vi "test reset.vi"   [LabVIEW 2018]
uses:
  <vilib>/rvi/interface/nirviReadWriteControl/nirviReadWriteControl.xnode
  <vilib>/rvi/interface/Simulation/niFpgaSimulationCallBeginRW.vi
  <vilib>/rvi/errors/niLvFpgaAdjustHostInterfaceError.vi
  <vilib>/rvi/interface/nirviOpenFPGA/nirviOpenFPGA.xnode
  NiFpgaLv.dll
  <vilib>/Utility/error.llb/Error Cluster From Error Code.vi
  FPGA Bitfiles/Dentalrobot_FPGATarget_1DIOBoardTestFPG_3A5PBD8+om0.lvbitx
  FPGA/FPGA_Dental robot.vi
  <vilib>/FPGAPlugInAG/myRIO-1900/niLvFpga_Open_myRIO-1900.vi
  <vilib>/rvi/interface/common/dynamic/niFpgaDynamicAddResources.vi
  <vilib>/platform/TimedLoop/XDataNode/XDataNode.xnode
  <vilib>/Platform/TimedLoop/XDataNode/nitl_modes.ctl
  <vilib>/Platform/TimedLoop/XDataNode/XDNodeRunTimeDep.lvlib
  <vilib>/Platform/TimedLoop/XDataNode/wakeup.ctl
  <vilib>/Platform/TimedLoop/XDataNode/timing_clust.ctl
panel:
  # "Servor"
  # "Stepper"
types:
  T1 = typedef "XDNodeRunTimeDep.lvlib/timing_clust.ctl" = cluster{"Expected End [f-1]":u64, "Actual End [f-1]":u64, "Finished Late? [f-1]":bool, "Expected End [i-1]":u64, "Actual End [i-1]":u64, "Finished Late? [i-1]":bool, "Expected Start [i]":u64, "Actual Start [i]":u64, "Expected Start [f]":u64, "Actual Start [f]":u64, "Source Name":string, "Structure Name":string, "Period":i64, "Deadline":i64, "Offset":i64, "Start":i64, "Priority":i32, "Timeout":i32, "Mode":T2, "Wakeup Reason":T3, "Error":errorcluster, "Source Type":string, "Secondary Source Type":string, "Global End Time":u64, "Global Start Time":u64, "Frame Duration":u64, "Iteration Duration":u64, "Assigned CPU":i32, "I/O Scan Engine Mode":u32}
  T2 = typedef "XDNodeRunTimeDep.lvlib/nitl_modes.ctl" = enum32{"No Change", "Process missed periods, maintain original phase", "Discard missed periods, maintain original phase", "Process missed periods, ignore original phase", "Discard missed periods, ignore original phase"}
  T3 = typedef "XDNodeRunTimeDep.lvlib/wakeup.ctl" = enum32{"Normal", "Aborted", "Asynchronous wakeup", "Timing source error", "Timed loop error", "Timeout"}
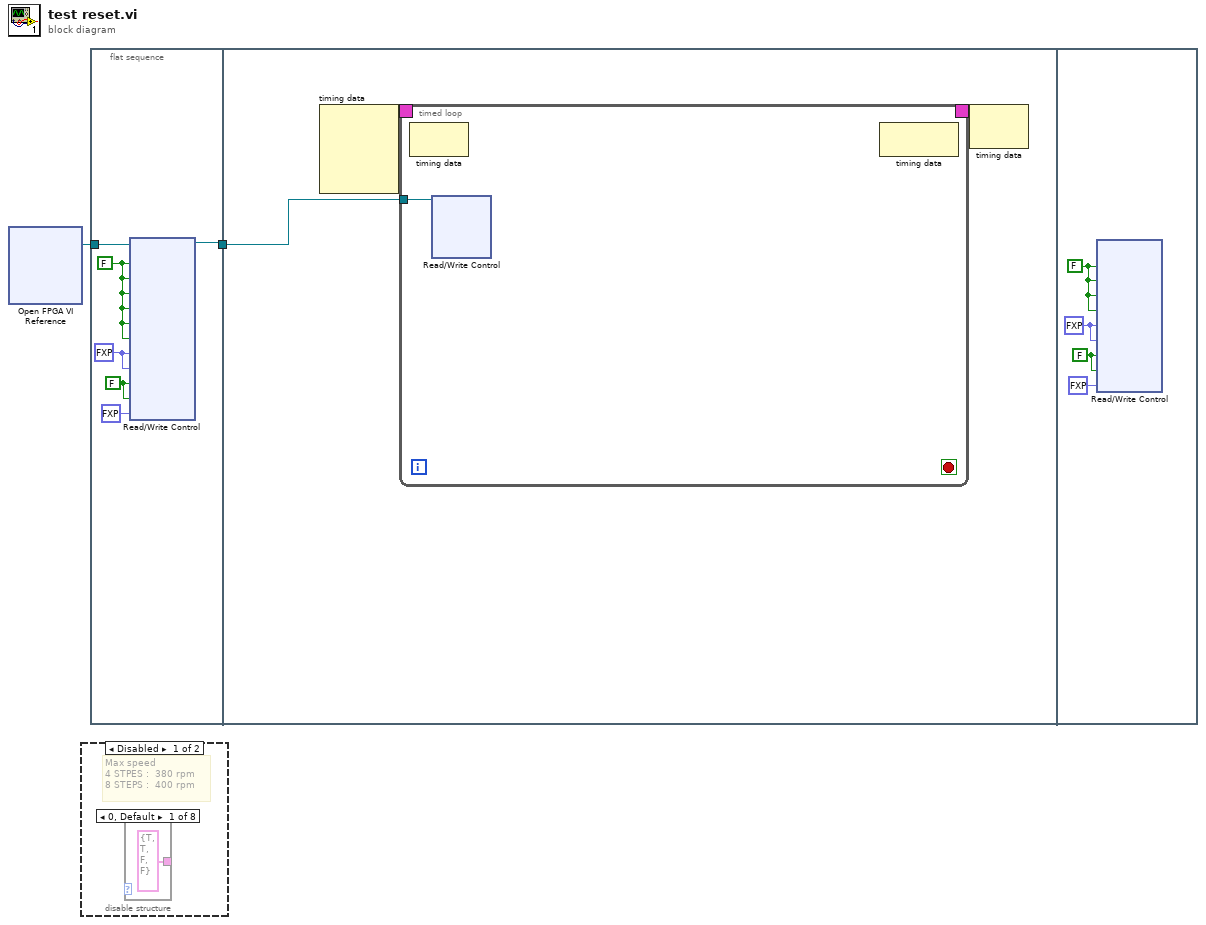
[diagram p0: block diagram]
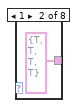
[diagram p2: hidden frame]
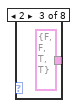
[diagram p3: hidden frame]
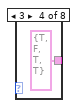
[diagram p4: hidden frame]
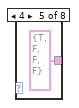
[diagram p5: hidden frame]
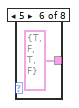
[diagram p6: hidden frame]
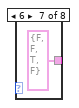
[diagram p7: hidden frame]
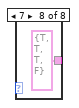
[diagram p8: hidden frame]
diagram:
  n1 = xnode "Open FPGA VI Reference"() -> ("FPGA VI Reference Out"=w1:refnum<k20>)  [unwired: 2 in, 1 out]
  n2 = disable-structure shown="Disabled" {
    frame Disabled {
      # "Max speed\n4 STPES :  380 rpm\n8 STEPS :  400 rpm"
      n3 = case shown="0, Default" {
        selector: _ -> [_ _ w6 _ _ _ _ _]
        tunnel: [cluster{bool, bool, bool, bool} {TRUE, TRUE, FALSE, FALSE} cluster{bool, bool, bool, bool} {TRUE, TRUE, TRUE, TRUE} cluster{bool, bool, bool, bool} {FALSE, FALSE, TRUE, TRUE} cluster{bool, bool, bool, bool} {TRUE, FALSE, TRUE, TRUE} cluster{bool, bool, bool, bool} {TRUE, FALSE, FALSE, FALSE} cluster{bool, bool, bool, bool} {TRUE, FALSE, TRUE, FALSE} cluster{bool, bool, bool, bool} {FALSE, FALSE, TRUE, FALSE} cluster{bool, bool, bool, bool} {TRUE, TRUE, TRUE, FALSE}] -> _
        frame 0, Default {
        }
        frame 1 {
        }
        frame 2 {
        }
        frame 3 {
        }
        frame 4 {
        }
        frame 5 {
        }
        frame 6 {
        }
        frame 7 {
        }
      }
    }
    frame Enabled {
    }
  }
  n4 = flat-sequence {
    tunnel: [w16] -> w2
    tunnel: w1 -> [w14]
    tunnel: w2 -> [w18]
    frame #0 {
      w12 = FALSE ("ENA4")
      w15 = fxp<+,32,0> 0.0 ("CH1 DC")
      w17 = FALSE ("ENA1")
      n5 = xnode "Read/Write Control"("FPGA VI Reference In"=w14, "ENA1"=w17, "STBY1"=w17, "DIR1"=w17, "ENA2"=w17, "STBY2"=w17, "DIR2"=w17, "CH1 DC"=w15, "CH2 DC"=w15, "ENA4"=w12, "STBY4"=w12, "CH4 DC"=fxp<+,32,0> 0.0) -> ("FPGA VI Reference Out"=w16:refnum<k20>)  [unwired: 1 in, 1 out]
    }
    frame #1 {
      n6 = node-c288() -> (w20:T1)  [unwired: 4 in]
      n7 = timed-loop {
        timing: w20 -> [_]
        timing-out: [_] -> w19
        tunnel: w18 -> [w21]
        stop <- _ stop-if-true
        n8 = node-c288() -> ()  [unwired: 1 in, 1 out]
        n9 = xnode "Read/Write Control"("FPGA VI Reference In"=w21) -> ()  [unwired: 4 in, 2 out]
        n10 = node-c288() -> ()  [unwired: 1 in, 1 out]
      }
      n11 = node-c288(w19) -> ()  [unwired: 1 out]
    }
    frame #2 {
      w27 = FALSE ("ENA4")
      w28 = fxp<+,32,0> 0.0 ("CH1 DC")
      w29 = FALSE ("ENA1")
      n12 = xnode "Read/Write Control"("ENA1"=w29, "STBY1"=w29, "ENA2"=w29, "STBY2"=w29, "CH1 DC"=w28, "CH2 DC"=w28, "ENA4"=w27, "STBY4"=w27, "CH4 DC"=fxp<+,32,0> 0.0) -> ()  [unwired: 2 in, 2 out]
    }
  }
